vi "HTML Report Numeric Tag Attributes.vi"(4 "default value (0)":i32, 5 "values":i32[](array[numeric]), 6 "labels":string[](array[string]), 7 "tag attributes in":string) -> (3 "tag attributes out":string)   [LabVIEW 2020, in "NI_ReportGenerationCore.lvlib"]
doc: "For non-default values, constructs the appropriate attributes."
uses:
  <vilib>/Utility/NIReport.llb/NI_ReportGenerationCore.lvlib
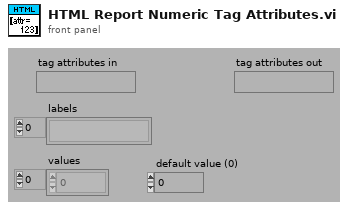
[diagram p1: front panel]
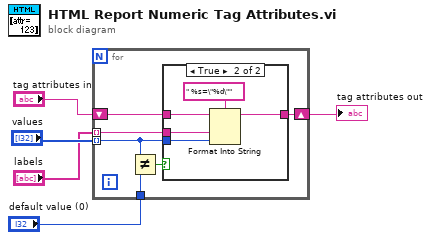
[diagram p0: block diagram]
diagram:
  n1 = for {
    shift-right: [w10] -> w3
    shift-left: "tag attributes in" -> [w11]
    tunnel: "values" -> [w8] mode=indexing
    tunnel: "labels" -> [w9] mode=indexing
    tunnel: "default value (0)" -> [w6]
    n2 = Not Equal?(x=w8, y=w6) -> (x != y?=w7:bool)
    n3 = case shown="True" w7 {
      tunnel: [w12 w17] -> w10
      tunnel: w11 -> [w12 w16]
      tunnel: w8 -> [_ w14]
      tunnel: w9 -> [_ w13]
      frame False {
      }
      frame True {
        n4 = Format Into String(format string=" %s=\"%d\"", initial string=w16, w13, w14) -> (resulting string=w17:string)  [unwired: 1 in, 1 out]
      }
    }
  }
  "tag attributes out" <- w3
